vi "add_duration.vi"   [LabVIEW 2016]
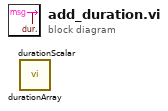
[diagram p0: block diagram]
diagram:
  n1 = call "durationArray.vi"() -> ()  [unwired: 5 in, 1 out]
  n2 = call "durationScalar.vi"() -> ()  [unwired: 5 in, 1 out]
